vi "Teleop.vi"(10 "Match Info":T1={"Autonomous Elapsed Seconds"=0.0, "TeleOp Elapsed Seconds"=28.6, "Disabled Elapsed Seconds"=17.195, "Visited Autonomous"=FALSE, "Visited TeleOp"=TRUE, "Visited Disabled"=TRUE, "Autonomous Settings"={"Autonomous Style"=enum."Independent", "VI Refnum"=refnum}}, 11 "Call Context":T2=enum."Stop") -> ()   [LabVIEW 2017]
doc: "This VI is called for each TeleOp packet received from the DS where the robot is not disabled. It is often used to read from the joysticks and update I/O or to update setpoints for timed control loops. It should complete and return within 20 milliseconds or it may miss DS packets."
uses:
  <vilib>/Rock Robotics/WPI/DriverStation/WPI_DriverStationDerivedRobotMode.ctl
  <vilib>/Rock Robotics/WPI/DriverStation/WPI_DriverStationMatch Info.ctl
  <vilib>/Rock Robotics/WPI/ThirdParty/Phoenix-LabVIEW/Motor Controller/Controls/CTRE_Phoenix_MotorControl_LimitSwitchSource_Local.ctl
  <vilib>/Rock Robotics/WPI/ThirdParty/Phoenix-LabVIEW/Motor Controller/Controls/CTRE_Phoenix_MotorControl_LimitSwitchNormal.ctl
  <vilib>/Rock Robotics/WPI/ThirdParty/Phoenix-LabVIEW/Motor Controller/Controls/CTRE_Phoenix_MotorControl_ControlMode.ctl
  <vilib>/Rock Robotics/WPI/Solenoid/WPI_SolenoidValue.ctl
  <vilib>/Rock Robotics/Network Tables/SD Read Boolean.vi
  <vilib>/Rock Robotics/Network Tables/SD Read Number.vi
  <vilib>/Rock Robotics/WPI/Utilities/WPI_GetSetVariantRefNum.vi
  Robot Global Data.vi
  <vilib>/Rock Robotics/WPI/Solenoid/WPI_SolenoidSetEnum.vi
panel:
  in  "Drive":enum16{"Cheesy", "Tank"}(ring)=enum."Tank"
  out "Sample Slider 0":dbl(slide) scale=0.0..5.0
  out "Sample Boolean 1":bool
  out "Sample Boolean 0":bool
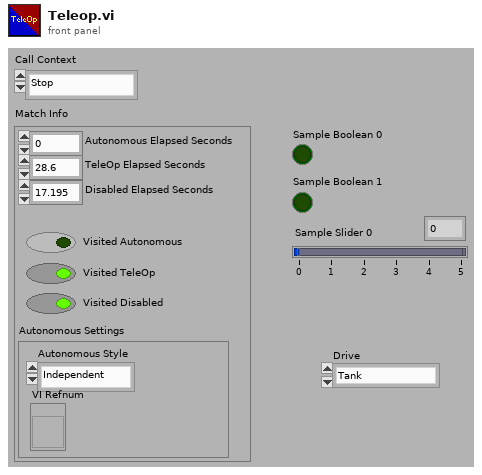
[diagram p1: front panel]
types:
  T1 = typedef "WPI_DriverStationMatch Info.ctl" = cluster{"Autonomous Elapsed Seconds":dbl, "TeleOp Elapsed Seconds":dbl, "Disabled Elapsed Seconds":dbl, "Visited Autonomous":bool, "Visited TeleOp":bool, "Visited Disabled":bool, "Autonomous Settings":cluster{"Autonomous Style":enum16{"Iterative", "Independent"}, "VI Refnum":refnum<vi>}}
  T2 = typedef "WPI_DriverStationDerivedRobotMode.ctl" = enum16{"Init", "Execute", "Stop"}
  T3 = typedef "CTRE_Phoenix_MotorControl_LimitSwitchNormal.ctl" = enum16{"Normally Open", "Normally Closed", "Disabled"}
  T4 = typedef "CTRE_Phoenix_MotorControl_LimitSwitchSource_Local.ctl" = enum16{"Feedback Connector", "Remote Talon SRX", "Remote CANifier", "Deactivated"}
  T5 = typedef "WPI_JoystickDevRef.ctl" = cluster{"Device":T6}
  T6 = typedef "WPI_JoystickDeviceEnum.ctl" = enum16{"USB 0", "USB 1", "USB 2", "USB 3", "USB 4", "USB 5"}
  T7 = typedef "WPI_RobotDriveDevRef.ctl" = cluster{"DevStatus":errorcluster, "Motors[]":T8[], "Square Inputs":bool, "Max Output":dbl}
  T8 = typedef "WPI_MotorControlDeviceRef.ctl" = cluster{"DeviceStatus":errorcluster, "Type":T9, "PWM":cluster{"PWM Channel":T10, "DeadBand":T11}, "CAN":cluster{"Device Number":u8, "SetOutput VI Ref":variant, "GetOutput VI Ref":variant, "Enable VI Ref":variant, "Disable VI Ref":variant, "Data":variant}, "Invert":bool, "DIO PWM":cluster{"PWM \"Enable\" Channel":T10, "DIOChannel":T12, "PWM Rate":dbl}}
  T9 = typedef "WPI_MotorControlType.ctl" = enum16{"PWM", "CAN", "DIO PWM"}
  T10 = typedef "FPGA_DIOPWMChannel.ctl" = enum8{"PWM 0", "PWM 1", "PWM 2", "PWM 3", "PWM 4", "PWM 5", "PWM 6", "PWM 7", "PWM 8", "PWM 9", "PWM MXP 0", "PWM MXP 1", "PWM MXP 2", "PWM MXP 3", "PWM MXP 4", "PWM MXP 5", "PWM MXP 6", "PWM MXP 7", "PWM MXP 8", "PWM MXP 9", "Invalid"}
  T11 = typedef "WPI_PWMDeadband.ctl" = cluster{"Name":string, "maxPositivePwm":i32, "minPositivePwm":i32, "centerPwm":i32, "maxNegativePwm":i32, "minNegativePwm":i32, "angularRange":u16}
  T12 = typedef "FPGA_DIOChannel.ctl" = enum8{"DIO 0", "DIO 1", "DIO 2", "DIO 3", "DIO 4", "DIO 5", "DIO 6", "DIO 7", "DIO 8", "DIO 9", "DIO MXP 0", "DIO MXP 1", "DIO MXP 2", "DIO MXP 3", "DIO MXP 4", "DIO MXP 5", "DIO MXP 6", "DIO MXP 7", "DIO MXP 8", "DIO MXP 9", "DIO MXP 10", "DIO MXP 11", "DIO MXP 12", "DIO MXP 13", "DIO MXP 14", "DIO MXP 15", "SPI Port CS1", "SPI Port CS2", "SPI Port CS3", "SPI Port MISO", "SPI Port MOSI", "Invalid"}
  T13 = typedef "WPI_PotentiometerDevRef.ctl" = cluster{"DevStatus":errorcluster, "Analog Channel":T14, "Invert Output":bool}
  T14 = typedef "FPGA_AIChannel.ctl" = enum8{"AI 0", "AI 1", "AI 2", "AI 3", "AI MXP 0", "AI MXP 1", "AI MXP 2", "AI MXP 3", "Invalid"}
  T15 = typedef "WPI_SolenoidValue.ctl" = enum16{"Off", "On", "Forward", "Reverse"}
  T16 = typedef "WPI_SolenoidDevRef.ctl" = cluster{"DevStatus":errorcluster, "Pneumatics Control Module":u8, "Forward Solenoid Channel":T17, "Reverse Solenoid Channel":T17}
  T17 = typedef "WPI_SolenoidChannel.ctl" = enum8{"Solenoid 0", "Solenoid 1", "Solenoid 2", "Solenoid 3", "Solenoid 4", "Solenoid 5", "Solenoid 6", "Solenoid 7", "Invalid"}
  T18 = typedef "CTRE_Phoenix_MotorControl_ControlMode.ctl" = u16
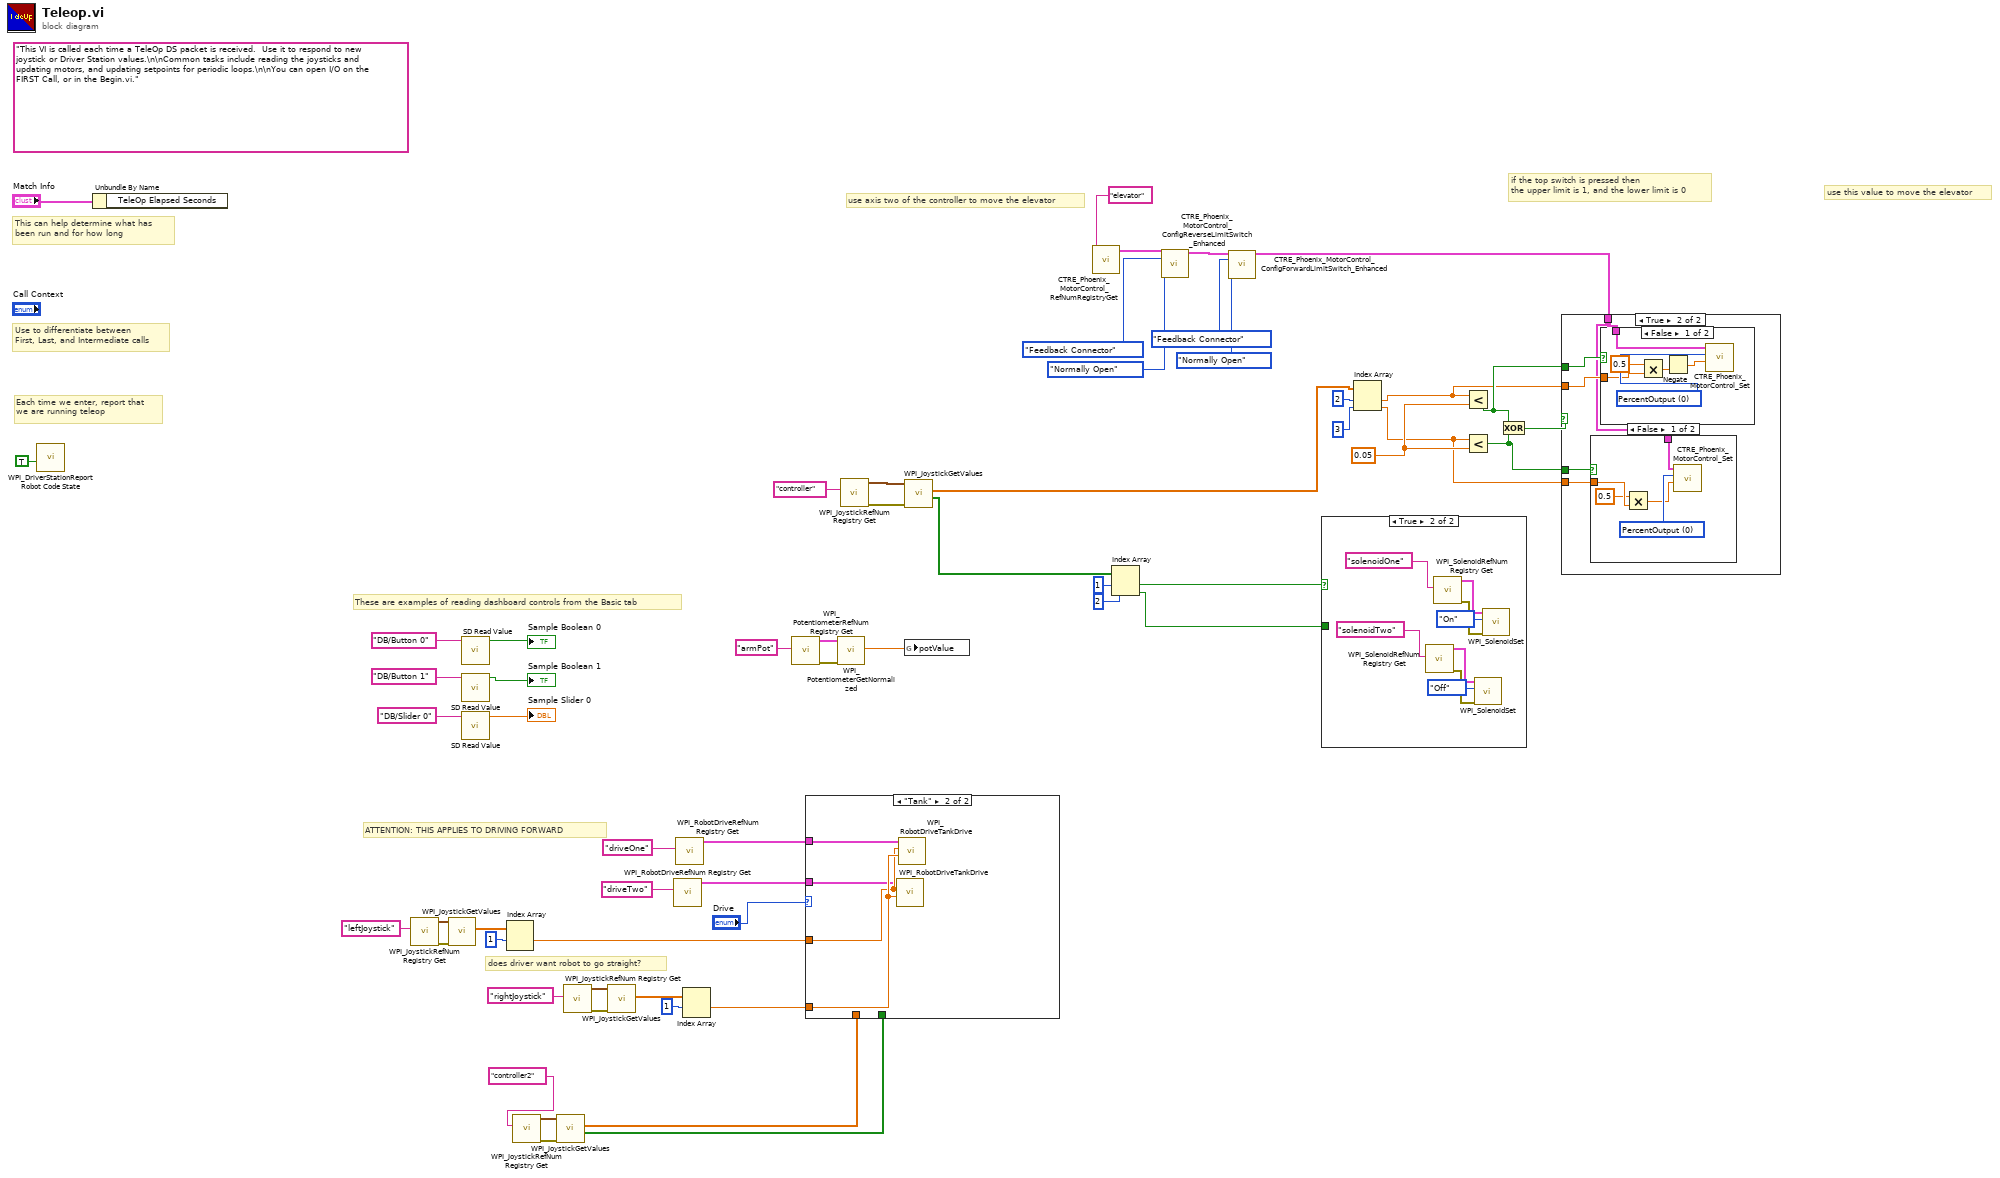
[diagram p0: block diagram]
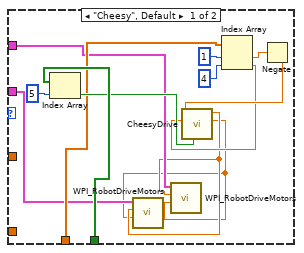
[diagram p2: hidden frame]
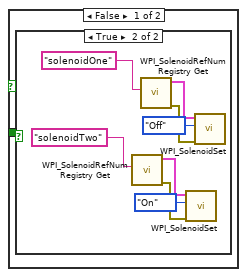
[diagram p3: hidden frame]
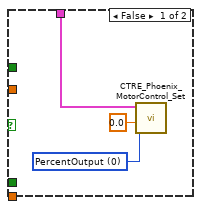
[diagram p5: hidden frame]
diagram:
  w19 = 0.05 ("x")
  (unwired) "This VI is called each time a TeleOp DS packet is received.  Use it to respond to new joystick or Driver Station values.\n\nCommon tasks include reading the joysticks and updating motors, and updating setpoints for periodic loops.\n\nYou can open I/O on the FIRST Call, or in the Begin.vi."
  # "ATTENTION: THIS APPLIES TO DRIVING FORWARD"
  # "does driver want robot to go straight?"
  # "use this value to move the elevator"
  # "if the top switch is pressed then\nthe upper limit is 1, and the lower limit is 0"
  # "use axis two of the controller to move the elevator"
  # "These are examples of reading dashboard controls from the Basic tab"
  # "Each time we enter, report that\nwe are running teleop"
  # "Use to differentiate between\nFirst, Last, and Intermediate calls"
  # "This can help determine what has\nbeen run and for how long"
  n1 = call <vilib>:"WPI_DriverStationReport Robot Code State.vi"("TeleOp"=TRUE ("Autonomous")) -> ()  [unwired: 10 in, 1 out]
  n2 = Unbundle By Name("Match Info") -> ()  [unwired: 1 out]
  n3 = call <vilib>:"WPI_JoystickRefNum Registry Get.vi"("refnum name"="leftJoystick") -> ("error out"=w40:errorcluster, "JoystickDevRef"=w39:T5)  [unwired: 9 in]
  n4 = call <vilib>:"WPI_JoystickGetValues.vi"("error in (no error)"=w40, "JoystickDevRef"=w39) -> ("Axes"=w37:dbl[])  [unwired: 5 in, 4 out]
  n5 = call-poly <vilib>:"SD Read Value.vi"("Name"="DB/Button 0" ("refnum name")) -> ("Boolean"=→"Sample Boolean 0":bool)  [unwired: 8 in, 2 out]
  n6 = call-poly <vilib>:"SD Read Value.vi"("Name"="DB/Button 1" ("refnum name")) -> ("Boolean"=→"Sample Boolean 1":bool)  [unwired: 8 in, 2 out]
  n7 = call-poly <vilib>:"SD Read Value.vi"("Name"="DB/Slider 0" ("refnum name")) -> ("Numeric"=→"Sample Slider 0":dbl)  [unwired: 8 in, 2 out]
  n8 = Index Array(array=w37, index #1=1 ("index")) -> (element #1=w24:dbl)  [unwired: 1 in, 1 out]
  n9 = call <vilib>:"WPI_JoystickRefNum Registry Get.vi"("refnum name"="controller2") -> ("error out"=w5:errorcluster, "JoystickDevRef"=w6:T5)  [unwired: 9 in]
  n10 = call <vilib>:"WPI_JoystickGetValues.vi"("error in (no error)"=w5, "JoystickDevRef"=w6) -> ("Buttons"=w1:bool[], "Axes"=w2:dbl[])  [unwired: 5 in, 3 out]
  n11 = call <vilib>:"WPI_JoystickRefNum Registry Get.vi"("refnum name"="rightJoystick") -> ("error out"=w43:errorcluster, "JoystickDevRef"=w42:T5)  [unwired: 9 in]
  n12 = call <vilib>:"WPI_JoystickGetValues.vi"("error in (no error)"=w43, "JoystickDevRef"=w42) -> ("Axes"=w38:dbl[])  [unwired: 5 in, 4 out]
  n13 = call <vilib>:"WPI_RobotDriveRefNum Registry Get.vi"("refnum name"="driveTwo") -> ("RobotDriveDevRef"=w23:T7)  [unwired: 9 in, 1 out]
  n14 = call <vilib>:"WPI_RobotDriveRefNum Registry Get.vi"("refnum name"="driveOne") -> ("RobotDriveDevRef"=w22:T7)  [unwired: 9 in, 1 out]
  n15 = Index Array(array=w38, index #1=1 ("index")) -> (element #1=w25:dbl)  [unwired: 1 in, 1 out]
  n16 = call <vilib>:"WPI_PotentiometerRefNum Registry Get.vi"("refnum name"="armPot") -> ("error out"=w48:errorcluster, "PotDevRef"=w47:T13)  [unwired: 9 in]
  n17 = case shown="\"Tank\"" "Drive" {
    tunnel: w25 -> [_ w76]
    tunnel: w24 -> [_ w75]
    tunnel: w23 -> [w62 w74]
    tunnel: w22 -> [w63 w73]
    tunnel: w2 -> [w66 _]
    tunnel: w1 -> [w68 _]
    frame "Cheesy", Default {
      n18 = Index Array(array=w68, index=5) -> (element=w67:bool)
      n19 = Index Array(array=w66, index #1=1 ("index"), index #2=4 ("index")) -> (element #1=w69:dbl, element #2=w64:dbl)
      n20 = Negate(x=w69) -> (-x=w65:dbl)
      n21 = call "CheesyDrive.vi"("Quickturn"=w67, "Wheel"=w64, "Throttle"=w65) -> ("Right PWM"=w60:dbl, "Left PWM"=w61:dbl)  [unwired: 7 in]
      n22 = call <vilib>:"WPI_RobotDriveMotors.vi"("RightSpeed"=w60, "LeftSpeed"=w61, "RobotDriveDevRef"=w62) -> ()  [unwired: 1 in, 8 out]
      n23 = call <vilib>:"WPI_RobotDriveMotors.vi"("RightSpeed"=w60, "LeftSpeed"=w61, "RobotDriveDevRef"=w63) -> ()  [unwired: 1 in, 8 out]
    }
    frame "Tank" {
      n24 = call <vilib>:"WPI_RobotDriveTankDrive.vi"("Right axis value"=w76, "Left axis value"=w75, "RobotDriveDevRef"=w74) -> ()  [unwired: 6 in, 3 out]
      n25 = call <vilib>:"WPI_RobotDriveTankDrive.vi"("Right axis value"=w76, "Left axis value"=w75, "RobotDriveDevRef"=w73) -> ()  [unwired: 6 in, 3 out]
    }
  }
  n26 = call <vilib>:"WPI_PotentiometerGetNormalized.vi"("error in"=w48, "PotDevRef"=w47) -> ("Normalized Value"=w45:dbl)  [unwired: 7 in, 2 out]
  n27 = call <vilib>:"WPI_JoystickRefNum Registry Get.vi"("refnum name"="controller") -> ("error out"=w51:errorcluster, "JoystickDevRef"=w50:T5)  [unwired: 9 in]
  n28 = call <vilib>:"WPI_JoystickGetValues.vi"("error in (no error)"=w51, "JoystickDevRef"=w50) -> ("Buttons"=w11:bool[], "Axes"=w18:dbl[])  [unwired: 5 in, 3 out]
  n29 = global write "Robot Global Data.vi" "potValue"(w45) -> ()
  n30 = call <vilib>:"CTRE_Phoenix_MotorControl_RefNumRegistryGet.vi"("refnum name"="elevator") -> ("PhoenixMotorControlDevRef"=w31:T8)  [unwired: 9 in, 1 out]
  n31 = Index Array(array=w11, index #1=1 ("index"), index #2=2 ("index")) -> (element #1=w10:bool, element #2=w9:bool)
  n32 = call <vilib>:"CTRE_Phoenix_MotorControl_ConfigReverseLimitSwitch_Enhanced.vi"("PhoenixMotorControlDevRef"=w31, "Limit Switch Source"=CTRE_Phoenix_MotorControl_LimitSwitchSource_Local."Feedback Connector", "NormallyOpenOrClosed"=CTRE_Phoenix_MotorControl_LimitSwitchNormal."Normally Open") -> ("PhoenixMotorControlDevRef"=w36:T8)  [unwired: 11 in, 1 out]
  n33 = call <vilib>:"CTRE_Phoenix_MotorControl_ConfigForwardLimitSwitch_Enhanced.vi"("PhoenixMotorControlDevRef"=w36, "Limit Switch Source"=CTRE_Phoenix_MotorControl_LimitSwitchSource_Local."Feedback Connector", "NormallyOpenOrClosed"=CTRE_Phoenix_MotorControl_LimitSwitchNormal."Normally Open") -> ("PhoenixMotorControlDevRef"=w14:T8)  [unwired: 11 in, 1 out]
  n34 = case shown="True" w10 {
    tunnel: w9 -> [w77 _]
    frame False {
      n35 = case shown="True" w77 {
        frame False {
        }
        frame True {
          n36 = call <vilib>:"WPI_SolenoidRefNum Registry Get.vi"("refnum name"="solenoidTwo") -> ("error out"=w82:errorcluster, "SolenoidDevRef"=w84:T16)  [unwired: 9 in]
          n37 = call <vilib>:"WPI_SolenoidRefNum Registry Get.vi"("refnum name"="solenoidOne") -> ("error out"=w78:errorcluster, "SolenoidDevRef"=w80:T16)  [unwired: 9 in]
          n38 = call-poly <vilib>:"WPI_SolenoidSet.vi"("error in (no error)"=w82, "Value"=WPI_SolenoidValue."On", "SolenoidDevRef"=w84) -> ()  [unwired: 7 in, 2 out]
          n39 = call-poly <vilib>:"WPI_SolenoidSet.vi"("error in (no error)"=w78, "Value"=WPI_SolenoidValue."Off", "SolenoidDevRef"=w80) -> ()  [unwired: 7 in, 2 out]
        }
      }
    }
    frame True {
      n40 = call <vilib>:"WPI_SolenoidRefNum Registry Get.vi"("refnum name"="solenoidTwo") -> ("error out"=w89:errorcluster, "SolenoidDevRef"=w87:T16)  [unwired: 9 in]
      n41 = call <vilib>:"WPI_SolenoidRefNum Registry Get.vi"("refnum name"="solenoidOne") -> ("error out"=w93:errorcluster, "SolenoidDevRef"=w91:T16)  [unwired: 9 in]
      n42 = call-poly <vilib>:"WPI_SolenoidSet.vi"("error in (no error)"=w89, "Value"=WPI_SolenoidValue."Off", "SolenoidDevRef"=w87) -> ()  [unwired: 7 in, 2 out]
      n43 = call-poly <vilib>:"WPI_SolenoidSet.vi"("error in (no error)"=w93, "Value"=WPI_SolenoidValue."On", "SolenoidDevRef"=w91) -> ()  [unwired: 7 in, 2 out]
    }
  }
  n44 = Index Array(array=w18, index #1=2 ("index"), index #2=3 ("index")) -> (element #1=w13:dbl, element #2=w12:dbl)
  n45 = Less?(x=w13, y=w19) -> (x < y?=w15:bool)
  n46 = Less?(x=w12, y=w19) -> (x < y?=w16:bool)
  n47 = Exclusive Or(1:w16, 2:w15) -> (0:w17:bool)
  n48 = case shown="True" w17 {
    tunnel: w16 -> [_ w101]
    tunnel: w15 -> [_ w100]
    tunnel: w14 -> [w94 w97]
    tunnel: w13 -> [_ w99]
    tunnel: w12 -> [_ w98]
    frame False {
      w95 = T18 0 items=["PercentOutput"=0, "Position"=1, "Velocity"=2, "Current"=3, "Follower"=5, "MotionProfile"=6, "MotionMagic"=7, "MotionMagicArc"=8, "MotionProfileArc"=10, "Disabled"=15] ("Control Mode")
      n49 = call <vilib>:"CTRE_Phoenix_MotorControl_Set.vi"("Output"=0.0, "Control Mode"=w95, "PhoenixMotorControlDevRef"=w94) -> ()  [unwired: 7 in, 2 out]
    }
    frame True {
      n50 = case shown="False" w101 {
        tunnel: w98 -> [w104 _]
        tunnel: w97 -> [w102 _]
        frame False {
          w106 = T18 0 items=["PercentOutput"=0, "Position"=1, "Velocity"=2, "Current"=3, "Follower"=5, "MotionProfile"=6, "MotionMagic"=7, "MotionMagicArc"=8, "MotionProfileArc"=10, "Disabled"=15] ("Control Mode")
          n51 = Multiply(x=0.5, y=w104) -> (x*y=w105:dbl)
          n52 = call <vilib>:"CTRE_Phoenix_MotorControl_Set.vi"("Output"=w105, "Control Mode"=w106, "PhoenixMotorControlDevRef"=w102) -> ()  [unwired: 7 in, 2 out]
        }
        frame True {
        }
      }
      n53 = case shown="False" w100 {
        tunnel: w97 -> [w111 _]
        tunnel: w99 -> [w109 _]
        frame False {
          w112 = T18 0 items=["PercentOutput"=0, "Position"=1, "Velocity"=2, "Current"=3, "Follower"=5, "MotionProfile"=6, "MotionMagic"=7, "MotionMagicArc"=8, "MotionProfileArc"=10, "Disabled"=15] ("Control Mode")
          n54 = Multiply(x=0.5, y=w109) -> (x*y=w108:dbl)
          n55 = Negate(x=w108) -> (-x=w110:dbl)
          n56 = call <vilib>:"CTRE_Phoenix_MotorControl_Set.vi"("Output"=w110, "Control Mode"=w112, "PhoenixMotorControlDevRef"=w111) -> ()  [unwired: 7 in, 2 out]
        }
        frame True {
        }
      }
    }
  }
